vi "Export Table.vi"(8 "error in (no error)":errorcluster, 11 "Report Viewer in":refnum<class "Report Viewer.lvclass">) -> (0 "error out":errorcluster, 3 "Report Viewer out":refnum<class "Report Viewer.lvclass">)   [LabVIEW 2019, in "Report Viewer.lvlib" / "Report Viewer.lvclass"]
uses:
  Library/Report Viewer.lvclass
  Library/Report Viewer.lvclass/Report Viewer.ctl
  <vilib>/Utility/file.llb/Write Delimited Spreadsheet (string).vi
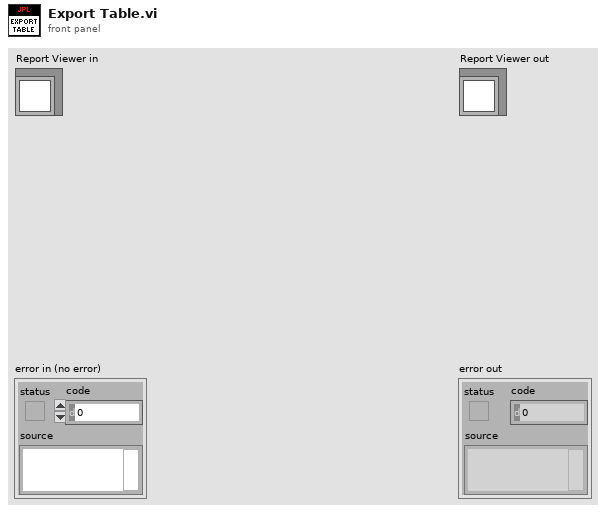
[diagram p1: front panel]
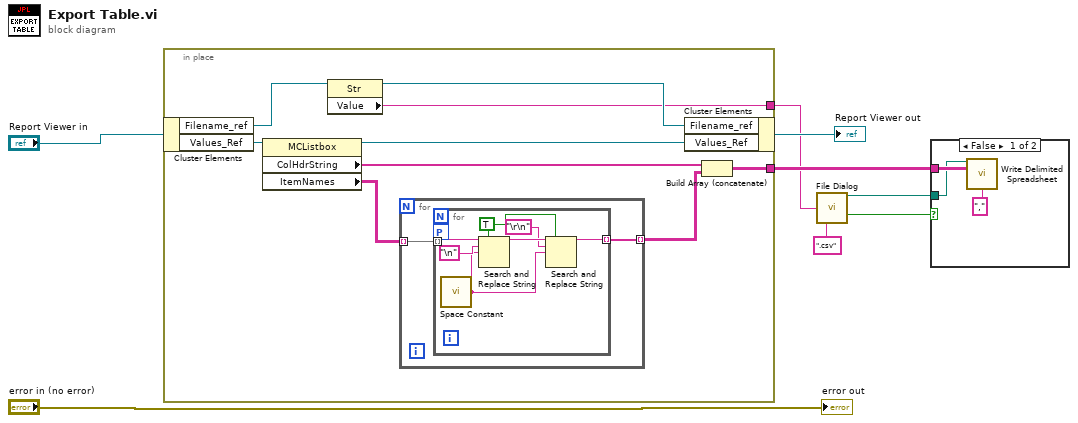
[diagram p0: block diagram]
diagram:
  n1 = in-place {
    in-place-border: [w14] -> w5
    in-place-border: [w9] -> w1
    n2 = in-place-cluster #1("Report Viewer in") -> ("Filename_ref"=w11:refnum<vi>, "Values_Ref"=w17:refnum<vi>)
    n3 = property class="MCListbox"(reference=w17) -> (reference out=w16:refnum<vi>, "ColHdrString"=w15:string[], "ItemNames"=w13:string[][])  [unwired: 1 in, 1 out]
    n4 = property class="Str"(reference=w11) -> (reference out=w10:refnum<vi>, "Value"=w9:string)  [unwired: 1 in, 1 out]
    n5 = for {
      tunnel: w13 -> [w19] mode=indexing
      tunnel: [w18] -> w12 mode=indexing
      n6 = for {
        tunnel: w19 -> [w26] mode=indexing
        tunnel: [w23] -> w18 mode=indexing
        workers-P: _ -> [_]
        w20 = TRUE ("replace all? (F)")
        n7 = call <vilib>:"Space Constant.vi"() -> ("String"=w22:string)
        n8 = Search and Replace String(replace all?=w20, input string=w26, search string="\n", replace string=w22) -> (result string=w24:string)  [unwired: 4 in, 3 out]
        n9 = Search and Replace String(replace all?=w20, input string=w24, search string="\r\n", replace string=w22) -> (result string=w23:string)  [unwired: 4 in, 3 out]
      }
    }
    n10 = in-place-cluster #1("Filename_ref"=w10, "Values_Ref"=w16) -> (→"Report Viewer out":refnum<class "Report Viewer.lvclass">)
    n11 = Build Array (concatenate)(w15, w12) -> (w14:string[][])
  }
  n12 = call "File Dialog"("default name"=w1, "pattern (all files)"=".csv") -> ("selected path"=w2:path, "cancelled"=w3:bool)  [unwired: 10 in, 2 out]
  n13 = case shown="False" w3 {
    tunnel: w5 -> [w29 _]
    tunnel: w2 -> [w27 _]
    frame False {
      n14 = call-poly <vilib>:"Write Delimited Spreadsheet.vi"("file path (dialog if empty)"=w27, "2D data"=w29, "delimiter (\\t)"="," ("delimiter (\\t)")) -> ()  [unwired: 11 in, 2 out]
    }
    frame True {
    }
  }
  "error out" <- "error in (no error)"
